vi "enable_chop_acquisition - multi-channel with switch.vi"(8 "error in":errorcluster, 10 "rate (Hz)":dbl=1000.0 format="%#_13g") -> (0 "error out":errorcluster, 2 "Results":T1={"V ch0 Array"=[3.4835999979780263, 3.4836012242512018, 3.483602593669106, 3.483602875187073, 3.483603624311153, 3.4836014246538225, 3.4836000790933723, 3.483598690589504, 3.483600971362181, 3.4836009045613077, 3.4836017968301167, 3.483602183320884, 3.483601772972662, 3.483599630573223, 3.4835997928039153, 3.48360306127522, 3.4835999645775897, 3.483602603212088, 3.483601682314334, 3.4836016298279335, 3.4836007184731606, 3.483601085877964, 3.4836008186744705, 3.48360276067129, 3.483603972629993, 3.483602555497179, 3.4836040442023575, 3.4836005037560676, 3.4836012385656745, 3.4835983327276825, 3.4836000361499537, 3.4835996496591863], "V ch1 Array"=[3.484989779157926, 3.484986964411474, 3.4849895310785777, 3.4849928038176716, 3.484988009207191, 3.4849885769272375, 3.484984755551123, 3.4849849225276075, 3.484990389814783, 3.484991153135854, 3.4849909623055866, 3.4849907046847246, 3.4849919593937364, 3.4849831716598993, 3.4849891112519877, 3.484991687460605, 3.484991797188009, 3.4849885864687513, 3.4849866781660723, 3.4849856238288424, 3.4849856667656525, 3.4849869071623933, 3.484991301029312, 3.4849874080918473, 3.48499559471034, 3.4849913058000688, 3.484991172218881, 3.4849868642255832, 3.484988839318856, 3.484987689566492, 3.4849948552430514, 3.484990609269591], "V ch2 Array"=[3.4843205610753976, 3.484320284318311, 3.4843197308041387, 3.484322274106329, 3.484324001452282, 3.4843166149010796, 3.4843176074092517, 3.4843155889911905, 3.484317645582643, 3.484318623775793, 3.4843192631800957, 3.484319096171509, 3.484318337475359, 3.48431976897753, 3.4843188385011183, 3.4843182993019672, 3.4843183231603367, 3.4843167628229703, 3.48431954948053, 3.484316295198928, 3.4843157273697334, 3.484316295198928, 3.4843149305001915, 3.484317325880491, 3.4843121390709584, 3.484318709665923, 3.484318280215272, 3.484316829626405, 3.484318786012705, 3.484314563081301, 3.48431767898436, 3.484316738964601], "V ch3 Array"=[3.4815150809144653, 3.4815169223695444, 3.481518429881993, 3.4815154816456224, 3.4815139550507386, 3.4815120563483513, 3.481515796505817, 3.48151713704695, 3.4815146992657446, 3.4815155007280585, 3.481515896688607, 3.4815180625450988, 3.481515214491518, 3.4815130009289357, 3.48151500935533, 3.4815190929966455, 3.4815165168677784, 3.4815169032871083, 3.4815137308321145, 3.4815147088069627, 3.481516812645537, 3.481516745857011, 3.481518849695586, 3.4815143366994596, 3.4815162401724558, 3.481516569344478, 3.4815189928138564, 3.4815123759791553, 3.4815176856669865, 3.4815155150398853, 3.481519288591615, 3.4815183726346848], "V ch4 Array"=[3.4815150809144653, 3.4815169223695444, 3.481518429881993, 3.4815154816456224, 3.4815139550507386, 3.4815120563483513, 3.481515796505817, 3.48151713704695, 3.4815146992657446, 3.4815155007280585, 3.481515896688607, 3.4815180625450988, 3.481515214491518, 3.4815130009289357, 3.48151500935533, 3.4815190929966455, 3.4815165168677784, 3.4815169032871083, 3.4815137308321145, 3.4815147088069627, 3.481516812645537, 3.481516745857011, 3.481518849695586, 3.4815143366994596, 3.4815162401724558, 3.481516569344478, 3.4815189928138564, 3.4815123759791553, 3.4815176856669865, 3.4815155150398853, 3.481519288591615, 3.4815183726346848], "Elapsed Time (ms)"=1599, "DMM Fault Array"=[]})   [LabVIEW 2019]
doc: "This example demonstrates how to enable the Chop feature in a continuously acquire buffered voltage measurement using a DAQmx device.\n\nFor instructions on how to connect your signals to the DAQ device, refer to your device documentation."
uses:
  <instrlib>/niSwitch/niSwitch.llb/niSwitch Topologies.ctl
  OCVResults.ctl
  <instrlib>/niSwitch/niSwitch.llb/niSwitch Trigger Input.ctl
  <instrlib>/niSwitch/niSwitch.llb/niSwitch Scan Advanced Output.ctl
  <vilib>/DAQmx/read.llb/DAQmx Read (Analog 2D DBL NChan NSamp).vi
  <vilib>/DAQmx/create/channels.llb/DAQmx Create Channel (AI-Voltage-Basic).vi
  <vilib>/DAQmx/configure/timing.llb/DAQmx Timing (Sample Clock).vi
  <vilib>/DAQmx/miscellaneous.llb/DAQmx Fill In Error Info.vi
  <resource>/objmgr/daqmx.rc
panel:
  out "Elapsed Time (ms)":u32=1599
  in  "Type Def":T1={"V ch0 Array"=[3.4860192438984856, 3.4860191297168432, 3.4860192480889696, 3.486019388780445, 3.4860200552848166, 3.4860195698501135, 3.4860194367740833, 3.48601943363801, 3.4860193560307953, 3.4860188399429166, 3.486019346172368, 3.4860197228808754, 3.4860192492604813, 3.4860198681823347, 3.486019386629169, 3.486019609000733, 3.4860194222252203, 3.486019475094303, 3.4860195777883813, 3.4860198327972123, 3.4860194844791064, 3.4860192846597724, 3.486019604192855, 3.4860193890850635, 3.486019882549224, 3.4860193407836872, 3.486019819402258, 3.4860195718672933, 3.486019850290971, 3.486020065378193, 3.4860200812401376, 3.486019332827698, 3.486019539704669, 3.4860191856958327, 3.486019603338049, 3.4860197214840167, 3.4860195162856176, 3.486019661979488, 3.4860196152518625, 3.48601960972234, 3.486019510427399, 3.4860193955138996, 3.486019403923719, 3.4860191116981416, 3.486019283259686, 3.48601881184557, 3.4860196673230894, 3.486018902499217, 3.486019173963923, 3.486019332419299, 3.486019671202645, 3.486019499160391, 3.4860193137480726, 3.4860193110217956, 3.4860195130088014, 3.486019457464569, 3.486018832088054, 3.4860192806634824, 3.486019456596911, 3.4860193546431457, 3.486019205666364, 3.4860194794988364, 3.486019332920187, 3.4860189764454312, 3.4860194155707083, 3.486019464342129, 3.486019459378369, 3.4860192395365615, 3.486019018887167, 3.4860187312440396, 3.4860194234856827, 3.486019167144491, 3.486019322954545, 3.48601941556311, 3.486019112865338, 3.4860191373093796, 3.4860190631335772, 3.4860189837060633, 3.486019421078644, 3.4860195807691094, 3.486018781084102, 3.4860192815150843, 3.4860191116507178, 3.4860196897391127, 3.486019054482244, 3.4860193237434984, 3.4860194341181536, 3.486019107534501, 3.486019323345851, 3.486019194973677, 3.486019161730881, 3.486019175960558, 3.4860194881647844, 3.486019137883692, 3.4860194237810673, 3.486019240702601, 3.4860195063002863, 3.4860195279338497, 3.48601941521367, 3.4860192998594033], "V ch1 Array"=[3.4837635496144497, 3.4837633047078356, 3.483763519496143, 3.4837638386501917, 3.4837636749838783, 3.4837637622882767, 3.4837639960874567, 3.4837640653526893, 3.4837639002914216, 3.4837639948081716, 3.483764380840748, 3.4837637486370903, 3.4837636058739494, 3.4837640082997314, 3.4837639377349143, 3.483764152676197, 3.483764186328907, 3.483763658922308, 3.483763950595508, 3.483764349614305, 3.4837638707197667, 3.4837639694240075, 3.483763685524895, 3.4837640426104857, 3.483763773323028, 3.483763498861096, 3.48376386163464, 3.483763856182671, 3.4837637805094976, 3.483763376025008, 3.483763485394124, 3.483763737216476, 3.4837637488823647, 3.4837636870799384, 3.48376348307593, 3.4837637531514787, 3.4837640725319123, 3.4837636718839913, 3.4837640882494845, 3.483763595720128, 3.4837638710640184, 3.4837634353037403, 3.4837640127310228, 3.483763765786545, 3.483763965435208, 3.4837639356094123, 3.483763874493519, 3.4837639386973054, 3.483763836392622, 3.4837635278265235, 3.4837637173072933, 3.4837639264438756, 3.483763640566874, 3.483763106913948, 3.4837632637092986, 3.4837636505867873, 3.483763618410148, 3.483763671849778, 3.4837632178283666, 3.483763387233682, 3.483763281131254, 3.4837636013322024, 3.4837633057079733, 3.483763227327618, 3.4837634820027947, 3.4837631861156715, 3.483762983477066, 3.4837630334263046, 3.48376290875784, 3.483763232599418, 3.483762992554408, 3.4837626856166883, 3.4837631059287872, 3.483762813425183, 3.4837629087040725, 3.4837626099036934, 3.4837629622175927, 3.48376292288895, 3.4837632589985734, 3.483762886524989, 3.4837632610144427, 3.483762640667348, 3.4837627900286097, 3.4837628605073703, 3.4837625301098667, 3.483762589933555, 3.483762644047744, 3.4837630383446054, 3.4837628475429008, 3.4837633574684297, 3.4837628873032394, 3.4837626059584355, 3.483762748980832, 3.4837627125543214, 3.4837627065039456, 3.4837625152019323, 3.483762655577027, 3.4837625644890657, 3.483762586641063, 3.4837624149674027], "V ch2 Array"=[3.480869179811629, 3.4808692218497557, 3.480869138671519, 3.480869054699297, 3.480869011510365, 3.480869157197732, 3.4808692155328744, 3.480869471635288, 3.4808689594292206, 3.48086945076089, 3.480869460297174, 3.480869073256913, 3.4808692935975163, 3.4808692152632608, 3.4808692867089013, 3.4808692057176573, 3.4808687717598494, 3.4808694889465652, 3.4808697225710654, 3.4808695479967744, 3.4808689900519267, 3.4808689501574617, 3.4808694493861148, 3.480869392710721, 3.4808696704117006, 3.480869061775111, 3.480869230832857, 3.4808690498110715, 3.480869272251721, 3.480869182984733, 3.480868986153201, 3.4808695148516193, 3.480869285336756, 3.480869113289467, 3.480869321219842, 3.4808696853476415, 3.4808695734255553, 3.480869235137222, 3.480869247933297, 3.4808693725489355, 3.4808693970987883, 3.480869510249631, 3.480869077447023, 3.480869142955564, 3.480869810198066, 3.4808695210330862, 3.4808690281746526, 3.4808697940447284, 3.4808695256214586, 3.480869543704313, 3.4808695752111873, 3.4808694743349164, 3.480869402997512, 3.4808696440759235, 3.480869426102383, 3.480869437921433, 3.480869608329062, 3.4808695813646384, 3.480869231247081, 3.480869681482936, 3.4808696850419185, 3.480869147852085, 3.480869498009006, 3.480869210180875, 3.4808695475881706, 3.4808691625176307, 3.480869831997257, 3.4808697720708257, 3.4808697676147338, 3.4808693613028483, 3.480869321113382, 3.4808695723953145, 3.4808696503256313, 3.480869784646468, 3.4808693231656824, 3.480869815348858, 3.4808695842415895, 3.480870030556013, 3.4808698084316507, 3.480869756575092, 3.4808700398397106, 3.480869601892204, 3.4808695224207016, 3.480870206481561, 3.4808697521028567, 3.4808696686542224, 3.4808694863409126, 3.4808695575238113, 3.4808699065023303, 3.4808699638400196, 3.4808698631823836, 3.4808701101021295, 3.480869576271954, 3.4808697499119545, 3.480870271581758, 3.480869580700272, 3.4808700517526905, 3.4808702583002464, 3.4808700507095285, 3.480869823475541], "V ch3 Array"=[3.4846462570940635, 3.484646344612051, 3.484645744648206, 3.484645912481853, 3.4846463765223765, 3.4846459790344033, 3.484645991388148, 3.4846459949495276, 3.4846461321623687, 3.4846459792980466, 3.4846459502897926, 3.484645900398946, 3.484646406044855, 3.484646675084715, 3.4846462272866976, 3.484646061071726, 3.4846463560563388, 3.4846458628621204, 3.484646481637977, 3.484646699310659, 3.4846463490174218, 3.4846461232936154, 3.4846460582414216, 3.4846463570899213, 3.4846459057947308, 3.4846460556842596, 3.484646296030384, 3.4846460469738423, 3.48464658781997, 3.4846460245693365, 3.4846462795314737, 3.484646537085635, 3.4846463696141208, 3.4846462323319045, 3.4846461621354017, 3.484646601971744, 3.484646588329547, 3.484646695791384, 3.4846460264137344, 3.4846461593422626, 3.4846466656982935, 3.484646823450527, 3.484647012524444, 3.4846463505570626, 3.4846467729305797, 3.484646413280307, 3.48464649989975, 3.48464616810511, 3.4846465502016866, 3.4846468176917242, 3.484646635790896, 3.4846464989218693, 3.4846463465061155, 3.4846469659954202, 3.484647055263412, 3.484646589351149, 3.4846465424842292, 3.4846469626004875, 3.4846465155978295, 3.484646895602941, 3.4846462809210985, 3.4846465125913824, 3.4846467493560573, 3.4846468222999647, 3.4846468884980775, 3.4846465504399218, 3.4846466232460154, 3.484646653097931, 3.4846467313351366, 3.484646901512995, 3.4846468026062616, 3.4846468641960726, 3.4846469829861624, 3.4846471909486487, 3.484646883370365, 3.4846465532654762, 3.484647151525274, 3.484647178327674, 3.484646970005987, 3.4846469124260966, 3.4846470266927594, 3.484646758486475, 3.484646811518315, 3.484646952996467, 3.4846469195374183, 3.484647335077417, 3.4846469162977516, 3.484646966685987, 3.484646746192782, 3.4846472376848387, 3.4846470826060396, 3.484646707902158, 3.4846471664925933, 3.4846471496125684, 3.484646829256042, 3.4846473259364736, 3.484647176634124, 3.4846472224270593, 3.4846474931875475, 3.4846470047324956], "V ch4 Array"=[3.482921883101798, 3.48292201038743, 3.482921963650252, 3.48292232595166, 3.4829219295743936, 3.4829222500251023, 3.4829218631289827, 3.482921530631896, 3.4829218244984688, 3.4829222060011986, 3.482921953922925, 3.482922434358391, 3.4829218861123223, 3.4829224024812797, 3.482922119408693, 3.482921891932435, 3.482922097428749, 3.4829221620547077, 3.4829221751564283, 3.482922233556675, 3.4829222935528996, 3.482922460577868, 3.482922010835762, 3.4829223716134146, 3.4829219243006335, 3.482921971962534, 3.48292214332319, 3.4829226800188824, 3.482922110730465, 3.482922308133039, 3.4829222890143448, 3.4829218963348003, 3.4829222321373243, 3.4829224166371646, 3.482922437339793, 3.4829227251192765, 3.4829224629498805, 3.4829224981761575, 3.482922744640211, 3.482922055871053, 3.482922617234262, 3.4829224386727837, 3.4829223546749937, 3.4829226079428963, 3.4829226019926987, 3.482922626244296, 3.482923102428407, 3.4829225941259927, 3.482922684262713, 3.482922875117361, 3.482922843526534, 3.4829228813035367, 3.482922798160215, 3.4829228033313098, 3.482922729208571, 3.4829230463638323, 3.482923001878261, 3.4829225660015597, 3.4829227170501635, 3.482922912556587, 3.482923170700634, 3.482922745453038, 3.4829229565113202, 3.482922859113936, 3.482922615231731, 3.482923042810891, 3.482922931359675, 3.4829233142114684, 3.482922846410176, 3.482923004292494, 3.48292354951055, 3.482923184798173, 3.4829227918015793, 3.482923015660196, 3.4829232528293685, 3.4829227291783544, 3.4829230564932825, 3.482922959508547, 3.4829228878182956, 3.4829230996323073, 3.4829230305207095, 3.482922900213177, 3.482923542767866, 3.482923191269675, 3.4829231627478645, 3.482923425303535, 3.482923253521273, 3.482923128067224, 3.482923205492421, 3.4829229699938544, 3.482923351524313, 3.4829234043244677, 3.4829230246211997, 3.482923045679957, 3.4829234300085905, 3.4829232984556935, 3.4829235896745185, 3.482923548361324, 3.48292348716183, 3.482923770747649], "Elapsed Time (ms)"=11164, "DMM Fault Array"=[]}
  out "Measurement 4":dbl[](graph)=[3.4815150809144653, 3.4815169223695444, 3.481518429881993, 3.4815154816456224, 3.4815139550507386, 3.4815120563483513, 3.481515796505817, 3.48151713704695, 3.4815146992657446, 3.4815155007280585, 3.481515896688607, 3.4815180625450988, 3.481515214491518, 3.4815130009289357, 3.48151500935533, 3.4815190929966455, 3.4815165168677784, 3.4815169032871083, 3.4815137308321145, 3.4815147088069627, 3.481516812645537, 3.481516745857011, 3.481518849695586, 3.4815143366994596, 3.4815162401724558, 3.481516569344478, 3.4815189928138564, 3.4815123759791553, 3.4815176856669865, 3.4815155150398853, 3.481519288591615, 3.4815183726346848]
  out "Measurement 3":dbl[](graph)=[3.4843205610753976, 3.484320284318311, 3.4843197308041387, 3.484322274106329, 3.484324001452282, 3.4843166149010796, 3.4843176074092517, 3.4843155889911905, 3.484317645582643, 3.484318623775793, 3.4843192631800957, 3.484319096171509, 3.484318337475359, 3.48431976897753, 3.4843188385011183, 3.4843182993019672, 3.4843183231603367, 3.4843167628229703, 3.48431954948053, 3.484316295198928, 3.4843157273697334, 3.484316295198928, 3.4843149305001915, 3.484317325880491, 3.4843121390709584, 3.484318709665923, 3.484318280215272, 3.484316829626405, 3.484318786012705, 3.484314563081301, 3.48431767898436, 3.484316738964601]
  out "Measurement 2":dbl[](graph)=[3.484989779157926, 3.484986964411474, 3.4849895310785777, 3.4849928038176716, 3.484988009207191, 3.4849885769272375, 3.484984755551123, 3.4849849225276075, 3.484990389814783, 3.484991153135854, 3.4849909623055866, 3.4849907046847246, 3.4849919593937364, 3.4849831716598993, 3.4849891112519877, 3.484991687460605, 3.484991797188009, 3.4849885864687513, 3.4849866781660723, 3.4849856238288424, 3.4849856667656525, 3.4849869071623933, 3.484991301029312, 3.4849874080918473, 3.48499559471034, 3.4849913058000688, 3.484991172218881, 3.4849868642255832, 3.484988839318856, 3.484987689566492, 3.4849948552430514, 3.484990609269591]
  in  "# of Cells":i32=64
  in  "resource name":refnum<k15>="Switch" caption="Resource Name"
  in  "scan list":string="ch0->com0&ch16->com1;\n\n\n\n" caption="Scan List"
  in  "topology name":T2="2530/2-Wire Quad 16x1 Mux" caption="Topology Name"
  in  "Chop":bool=TRUE
  in  "Stop":bool
  out "Measurement":dbl[](graph)=[3.4835999979780263, 3.4836012242512018, 3.483602593669106, 3.483602875187073, 3.483603624311153, 3.4836014246538225, 3.4836000790933723, 3.483598690589504, 3.483600971362181, 3.4836009045613077, 3.4836017968301167, 3.483602183320884, 3.483601772972662, 3.483599630573223, 3.4835997928039153, 3.48360306127522, 3.4835999645775897, 3.483602603212088, 3.483601682314334, 3.4836016298279335, 3.4836007184731606, 3.483601085877964, 3.4836008186744705, 3.48360276067129, 3.483603972629993, 3.483602555497179, 3.4836040442023575, 3.4836005037560676, 3.4836012385656745, 3.4835983327276825, 3.4836000361499537, 3.4835996496591863]
  in  "Terminal Configuration":i32(ring)=10106 items=["default"=-1, "RSE"=10083, "NRSE"=10078, "Differential"=10106, "Pseudodifferential"=12529]
  in  "Max Voltage":dbl=10.0
  in  "Min Voltage":dbl=-10.0
  in  "Physical Channel":tag="4309/ai0:3"
  # "Switch Settings"
  # "DAQmx Settings"
  # "On (T)"
  # "Off (F)"
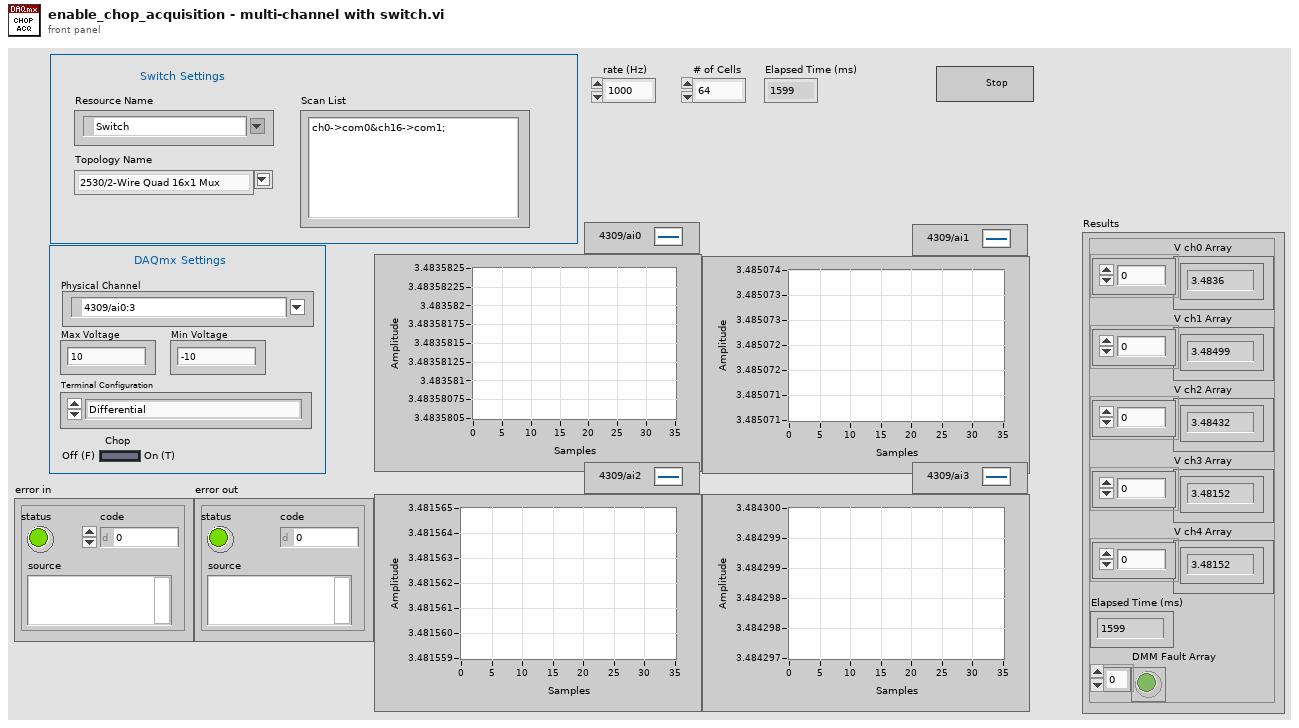
[diagram p1: front panel]
types:
  T1 = typedef "OCVResults.ctl" = cluster{"V ch0 Array":dbl[], "V ch1 Array":dbl[], "V ch2 Array":dbl[], "V ch3 Array":dbl[], "V ch4 Array":dbl[], "Elapsed Time (ms)":u32, "DMM Fault Array":bool[]}
  T2 = typedef "niSwitch Topologies.ctl" = string
  T3 = typedef "niSwitch Scan Advanced Output.ctl" = enum16{"None", "External", "TTL0", "TTL1", "TTL2", "TTL3", "TTL4", "TTL5", "TTL6", "TTL7", "ECL0", "ECL1", "PXI Star", "Rear Connector", "Front Connector", "Rear Connector Module 1", "Rear Connector Module 2", "Rear Connector Module 3", "Rear Connector Module 4", "Rear Connector Module 5", "Rear Connector Module 6", "Rear Connector Module 7", "Rear Connector Module 8", "Rear Connector Module 9", "Rear Connector Module 10", "Rear Connector Module 11", "Rear Connector Module 12", "Front Connector Module 1", "Front Connector Module 2", "Front Connector Module 3", "Front Connector Module 4", "Front Connector Module 5", "Front Connector Module 6", "Front Connector Module 7", "Front Connector Module 8", "Front Connector Module 9", "Front Connector Module 10", "Front Connector Module 11", "Front Connector Module 12"}
  T4 = typedef "niSwitch Trigger Input.ctl" = enum16{"Immediate", "External", "TTL0", "TTL1", "TTL2", "TTL3", "TTL4", "TTL5", "TTL6", "TTL7", "ECL0", "ECL1", "PXI Star", "Software Trigger Function", "Rear Connector", "Front Connector", "Rear Connector of Module 1", "Rear Connector of Module 2", "Rear Connector of Module 3", "Rear Connector of Module 4", "Rear Connector of Module 5", "Rear Connector of Module 6", "Rear Connector of Module 7", "Rear Connector of Module 8", "Rear Connector of Module 9", "Rear Connector of Module 10", "Rear Connector of Module 11", "Rear Connector of Module 12", "Front Connector of Module 1", "Front Connector of Module 2", "Front Connector of Module 3", "Front Connector of Module 4", "Front Connector of Module 5", "Front Connector of Module 6", "Front Connector of Module 7", "Front Connector of Module 8", "Front Connector of Module 9", "Front Connector of Module 10", "Front Connector of Module 11", "Front Connector of Module 12"}
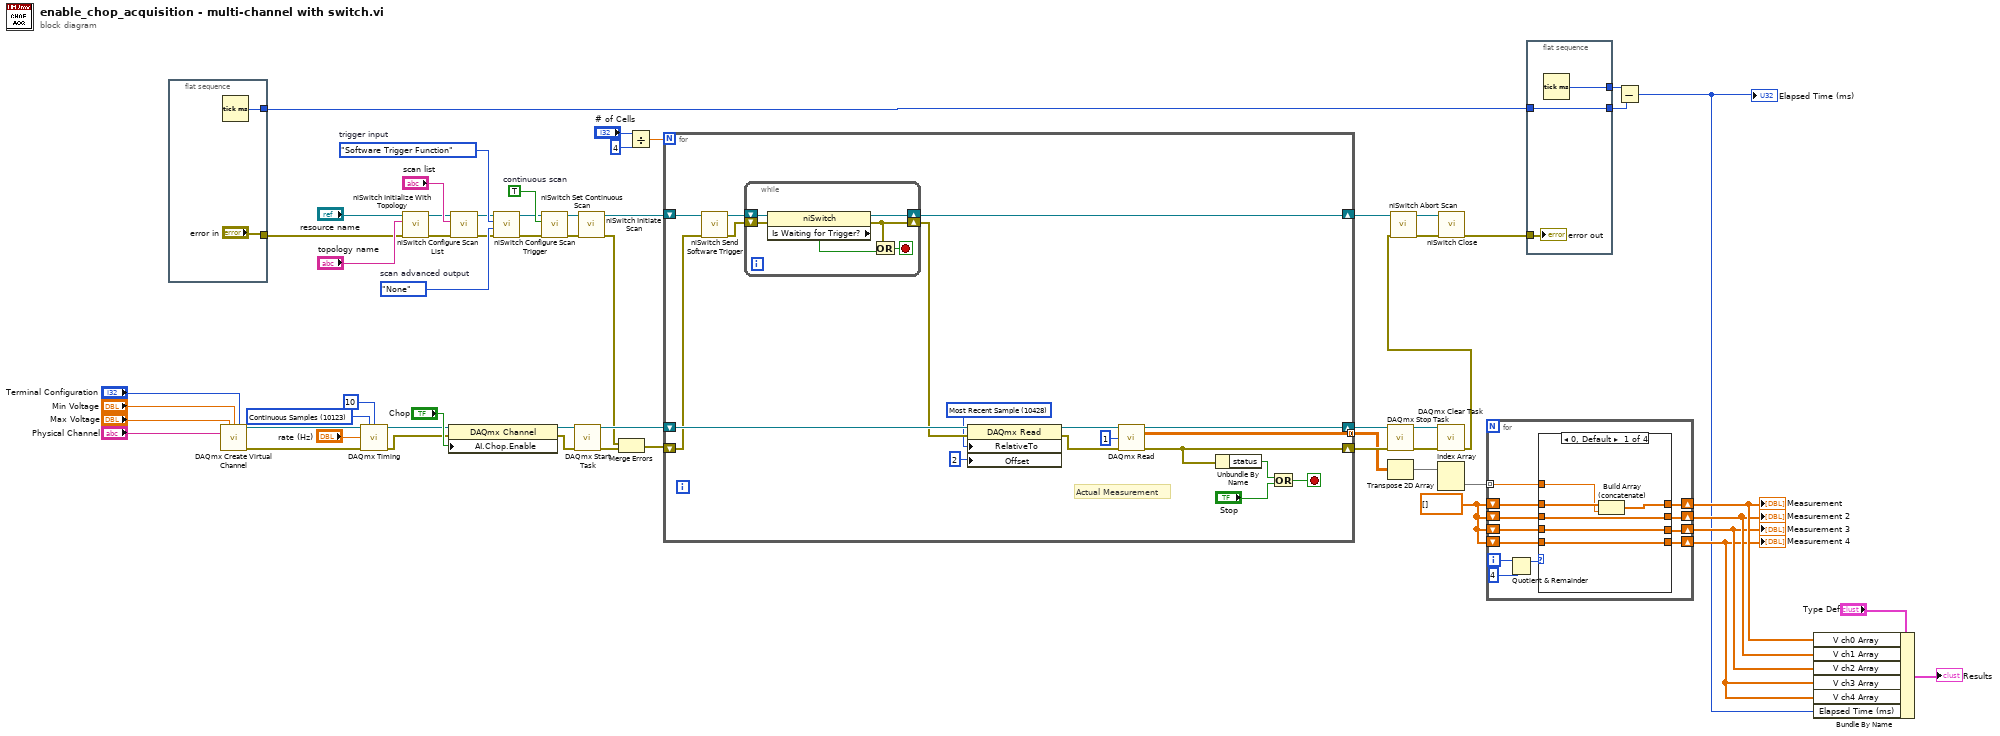
[diagram p0: block diagram]
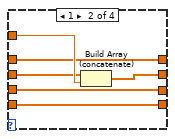
[diagram p2: hidden frame]
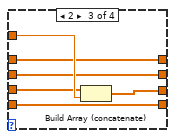
[diagram p3: hidden frame]
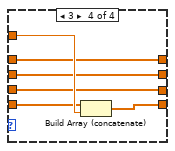
[diagram p4: hidden frame]
diagram:
  w20 = dbl[] [] ("History Data")
  w27 = 10123 items=["Finite Samples"=10178, "Continuous Samples"=10123, "Hardware Timed Single Point"=12522] ("sample mode")
  w52 = niSwitch_Scan_Advanced_Output."None"  # scan advanced output
  w51 = niSwitch_Trigger_Input."Software Trigger Function"  # trigger input
  w43 = TRUE  # continuous scan
  n1 = flat-sequence {
    tunnel: [w62] -> w14
    tunnel: ["error in"] -> w36
    frame #0 {
      n2 = Tick Count (ms)() -> (millisecond timer value=w62:u32)
    }
  }
  n3 = call-poly <vilib>:"DAQmx Create Virtual Channel.vi"("maximum value"="Max Voltage", "minimum value"="Min Voltage", "input terminal configuration"="Terminal Configuration", "physical channels"="Physical Channel") -> ("task out"=w32:refnum<k21>, "error out"=w35:errorcluster)  [unwired: 10 in]
  n4 = call-poly <vilib>:"DAQmx Timing.vi"("task/channels in"=w32, "sample mode"=w27, "samples per channel"=10, "rate"="rate (Hz)", "error in"=w35) -> ("task out"=w33:refnum<k21>, "error out"=w34:errorcluster)  [unwired: 9 in]
  n5 = call <instrlib>:"niSwitch Initialize With Topology.vi"("error in (no error)"=w36, "topology name"="topology name", "resource name"="resource name") -> ("error out"=w48:errorcluster, "instrument handle out"=w47:refnum<k15>)  [unwired: 2 in, 5 out]
  n6 = property class="DAQmx Channel"(reference=w33, error in=w34, "AI.Chop.Enable"="Chop") -> (reference out=w31:refnum<k21>, error out=w30:errorcluster)
  n7 = call <instrlib>:"niSwitch Configure Scan List.vi"("error in (no error)"=w48, "scan list"="scan list", "instrument handle"=w47) -> ("error out"=w41:errorcluster, "instrument handle out"=w39:refnum<k15>)  [unwired: 1 in, 6 out]
  n8 = call <instrlib>:"niSwitch Configure Scan Trigger.vi"("error in (no error)"=w41, "scan advanced output (External)"=w52, "trigger input (External)"=w51, "instrument handle"=w39) -> ("error out"=w42:errorcluster, "instrument handle out"=w38:refnum<k15>)  [unwired: 1 in, 5 out]
  n9 = call <instrlib>:"niSwitch Set Continuous Scan.vi"("error in (no error)"=w42, "continuous scan (False)"=w43, "instrument handle"=w38) -> ("error out"=w45:errorcluster, "instrument handle out"=w44:refnum<k15>)  [unwired: 7 out]
  n10 = call <vilib>:"DAQmx Start Task.vi"("task/channels in"=w31, "error in"=w30) -> ("task out"=w12:refnum<k21>, "error out"=w8:errorcluster)  [unwired: 12 in]
  n11 = call <instrlib>:"niSwitch Initiate Scan.vi"("error in (no error)"=w45, "instrument handle"=w44) -> ("error out"=w9:errorcluster, "instrument handle out"=w11:refnum<k15>)  [unwired: 8 out]
  n12 = Merge Errors(w9, w8) -> (w10:errorcluster)
  n13 = Divide(x="# of Cells", y=4) -> (x/y=w18:dbl)
  n14 = for {
    N: w18 -> [_]
    shift-right: [w72] -> w29
    shift-left: w11 -> [w79]
    shift-right: [w71] -> w25
    shift-left: w10 -> [w73]
    shift-right: [w75] -> w24
    shift-left: w12 -> [w77]
    tunnel: [w74] -> w23 mode=concatenating
    stop <- w78 stop-if-true
    w69 = 10428 items=["First Sample"=10424, "Current Read Position"=10425, "Reference Trigger"=10426, "First Pretrigger Sample"=10427, "Most Recent Sample"=10428] ("RelativeTo")
    # "Actual Measurement"
    n15 = call <instrlib>:"niSwitch Send Software Trigger.vi"("error in (no error)"=w73, "instrument handle"=w79) -> ("error out"=w66:errorcluster, "instrument handle out"=w67:refnum<k15>)  [unwired: 8 out]
    n16 = while {
      shift-right: [w84] -> w72
      shift-left: w67 -> [w86]
      shift-right: [w81] -> w70
      shift-left: w66 -> [w85]
      stop <- w83 stop-if-true
      n17 = property class="niSwitch"(reference=w86, error in=w85) -> (reference out=w84:refnum<k15>, error out=w81:errorcluster, "Is Waiting for Trigger?"=w82:bool)
      n18 = Or(x=w81, y=w82) -> (x .or. y?=w83:bool)
    }
    n19 = property class="DAQmx Read"(reference=w77, error in=w70, "RelativeTo"=w69, "Offset"=2) -> (reference out=w64:refnum<k21>, error out=w63:errorcluster)
    n20 = call-poly <vilib>:"DAQmx Read.vi"("task/channels in"=w64, "number of samples per channel"=1, "error in"=w63) -> ("task out"=w75:refnum<k21>, "data"=w74:dbl[][], "error out"=w71:errorcluster)  [unwired: 10 in]
    n21 = Unbundle By Name(w71) -> ("status"=w76:bool)
    n22 = Or(x=w76, y="Stop") -> (x .or. y?=w78:bool)
  }
  n23 = call <vilib>:"DAQmx Stop Task.vi"("task/channels in"=w24, "error in"=w25) -> ("task out"=w55:refnum<k21>, "error out"=w56:errorcluster)  [unwired: 12 in]
  n24 = Transpose 2D Array(2D array=w23) -> (transposed array=w22:dbl[][])
  n25 = call <vilib>:"DAQmx Clear Task.vi"("task in"=w55, "error in"=w56) -> ("error out"=w37:errorcluster)  [unwired: 13 in]
  n26 = call <instrlib>:"niSwitch Abort Scan.vi"("error in (no error)"=w37, "instrument handle"=w29) -> ("error out"=w46:errorcluster, "instrument handle out"=w40:refnum<k15>)  [unwired: 8 out]
  n27 = Index Array(array=w22) -> (element=w21:dbl[])  [unwired: 2 in]
  n28 = call <instrlib>:"niSwitch Close.vi"("error in (no error)"=w46, "instrument handle"=w40) -> ("error out"=w16:errorcluster)  [unwired: 9 out]
  n29 = for {
    tunnel: w21 -> [w95] mode=indexing
    shift-right: [w93] -> w6
    shift-left: w20 -> [w94]
    shift-right: [w92] -> w5
    shift-left: w20 -> [w91]
    shift-right: [w90] -> w4
    shift-left: w20 -> [w89]
    shift-right: [w88] -> w3
    shift-left: w20 -> [w87]
    i -> [w98]
    n30 = Quotient & Remainder(x=w98, y=4) -> (x-y*floor(x/y)=w96:i32)  [unwired: 1 out]
    n31 = case shown="0, Default" w96 {
      tunnel: w95 -> [w102 w110 w116 w122]
      tunnel: w94 -> [w103 w107 w113 w119]
      tunnel: [w104 w107 w113 w119] -> w93
      tunnel: [w101 w109 w112 w118] -> w92
      tunnel: w91 -> [w101 w108 w112 w118]
      tunnel: [w100 w106 w115 w117] -> w90
      tunnel: w89 -> [w100 w106 w114 w117]
      tunnel: [w99 w105 w111 w121] -> w88
      tunnel: w87 -> [w99 w105 w111 w120]
      frame 0, Default {
        n32 = Build Array (concatenate)(w103, w102) -> (w104:dbl[])
      }
      frame 1 {
        n33 = Build Array (concatenate)(w108, w110) -> (w109:dbl[])
      }
      frame 2 {
        n34 = Build Array (concatenate)(w114, w116) -> (w115:dbl[])
      }
      frame 3 {
        n35 = Build Array (concatenate)(w120, w122) -> (w121:dbl[])
      }
    }
  }
  "Measurement" <- w6
  "Measurement 2" <- w5
  "Measurement 3" <- w4
  "Measurement 4" <- w3
  n36 = flat-sequence {
    tunnel: w16 -> [w124]
    tunnel: [w125] -> w15
    tunnel: w14 -> [w123]
    tunnel: [w123] -> w13
    frame #0 {
      n37 = Tick Count (ms)() -> (millisecond timer value=w125:u32)
      "error out" <- w124
    }
  }
  n38 = Subtract(x=w15, y=w13) -> (x-y=w1:u32)
  "Elapsed Time (ms)" <- w1
  n39 = Bundle By Name(cluster="Type Def", "V ch0 Array"=w6, "V ch1 Array"=w5, "V ch2 Array"=w4, "V ch3 Array"=w3, "V ch4 Array"=w3, "Elapsed Time (ms)"=w1) -> (→"Results":T1)
